vi "Untitled 1.vi"() -> ()   [LabVIEW 2013]
uses:
  <vilib>/Analysis/6fits.llb/Curve Fitting Criteria.ctl
  <vilib>/Analysis/NI_AALPro.lvlib
panel:
  out "XY Graph 3":cluster{"Y":dbl[], "Y":dbl[]}[](graph)
  out "XY Graph 2":cluster{"X":dbl, "Y":dbl}[](graph)
  out "Array":cluster{dbl, dbl}[](array[cluster])
  out "XY Graph":cluster{"X":dbl, "Y":dbl}[](graph)
  in  "Pi/x":dbl
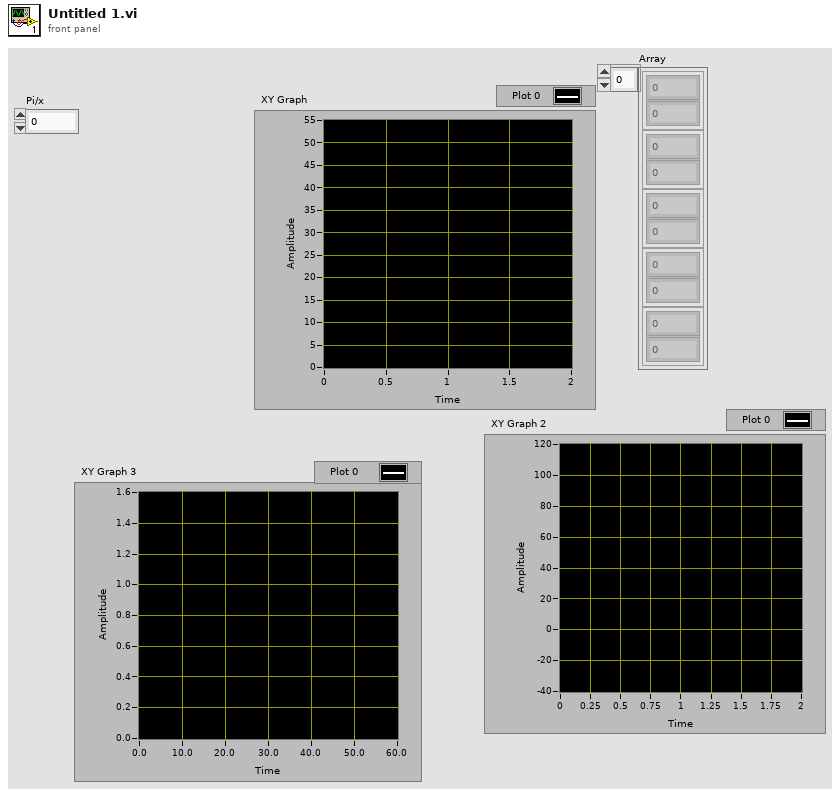
[diagram p1: front panel]
types:
  T1 = typedef "NI_AALPro.lvlib/Curve Fitting Criteria.ctl" = u16
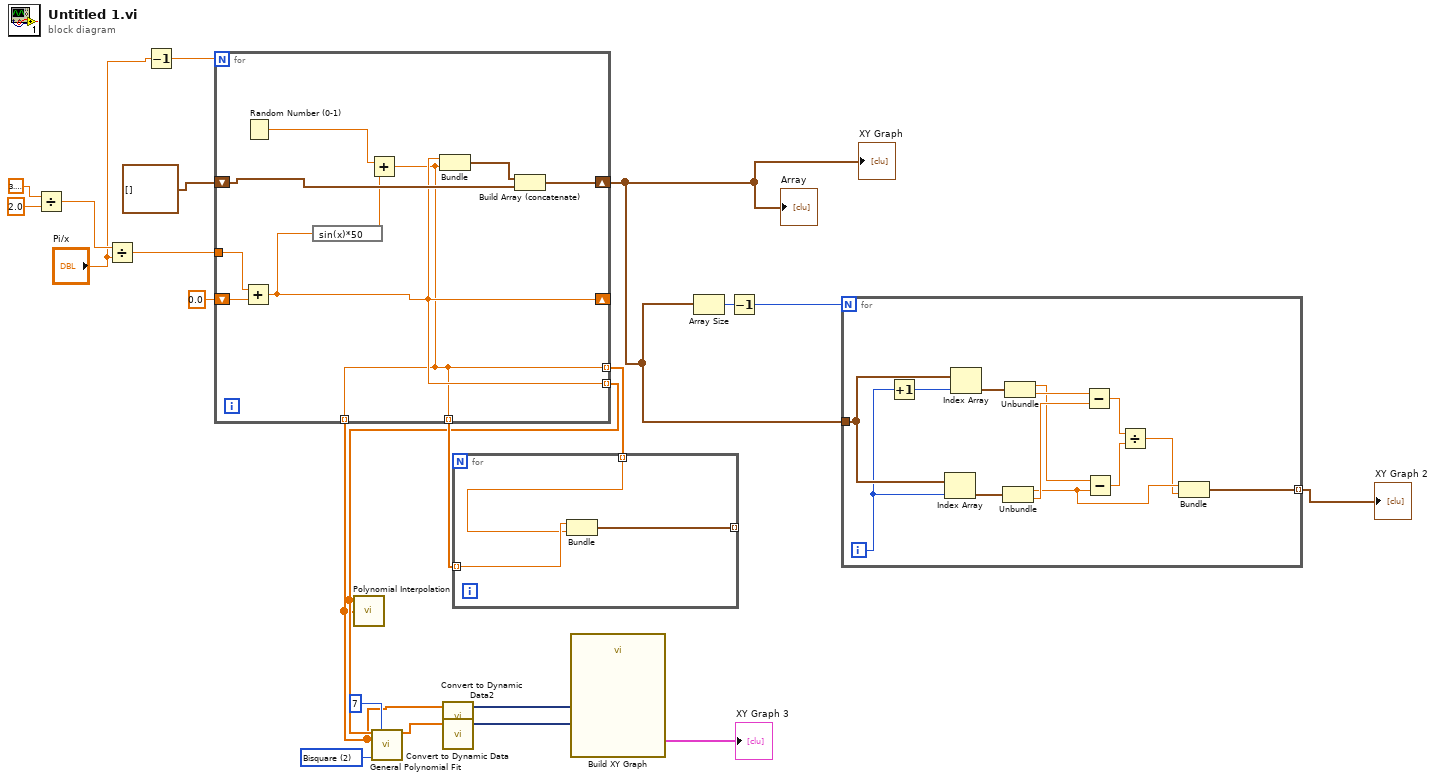
[diagram p0: block diagram]
diagram:
  w6 = T1 2 items=["Least Square", "Least Absolute Residual", "Bisquare"] ("method")
  n1 = Divide(x=3.141592653589793, y=2.0) -> (x/y=w19:dbl)
  n2 = Divide(x=w19, y="Pi/x") -> (x/y=w12:dbl)
  n3 = Decrement(x="Pi/x") -> (x-1=w16:dbl)
  n4 = for {
    N: w16 -> [_]
    tunnel: w12 -> [w31]
    shift-right: [w25] -> _
    shift-left: 0.0 -> [w30]
    shift-right: [w28] -> w1
    shift-left: cluster{dbl, dbl}[] [] -> [w27]
    tunnel: [w25] -> w7 mode=indexing
    tunnel: [w23] -> w4 mode=indexing
    tunnel: [w23] -> w2 mode=indexing
    tunnel: [w23] -> w8 mode=indexing
    n5 = Add(x=w31, y=w30) -> (x+y=w25:dbl)
    n6 = Random Number (0-1)() -> (number: 0 to 1=w24:dbl)
    n7 = expression code="sin(x)*50"(w25) -> (w26:dbl)
    n8 = Add(x=w24, y=w26) -> (x+y=w23:dbl)
    n9 = Bundle(w25, w23) -> (w29:cluster{dbl, dbl})  [unwired: 1 in]
    n10 = Build Array (concatenate)(w29, w27) -> (w28:cluster{dbl, dbl}[])
  }
  "XY Graph" <- w1
  "Array" <- w1
  n11 = call <vilib>:"Polynomial Interpolation.vi"("X"=w2, "Y"=w7) -> ()  [unwired: 1 in, 3 out]
  n12 = call <vilib>:"General Polynomial Fit.vi"("Y"=w7, "polynomial order"=7, "X"=w2, "method"=w6) -> ("Best Polynomial Fit"=w3:dbl[])  [unwired: 8 in, 3 out]
  n13 = call "Convert to Dynamic Data2"("Array"=w2) -> ("Dynamic Data Type"=w9:dynamicdata)  [unwired: 3 in]
  n14 = call "Convert to Dynamic Data"("Array"=w3) -> ("Dynamic Data Type"=w10:dynamicdata)  [unwired: 3 in]
  n15 = for {
    tunnel: w8 -> [w34] mode=indexing
    tunnel: [w33] -> _ mode=indexing
    tunnel: w4 -> [w32] mode=indexing
    n16 = Bundle(w34, w32) -> (w33:cluster{dbl, dbl})  [unwired: 1 in]
  }
  n17 = call "Build XY Graph"("Y Input"=w10, "X Input"=w9) -> ("XY Graph"=→"XY Graph 3":cluster{"X":dbl[], "Y":dbl[]}[])  [unwired: 8 in, 1 out]
  n18 = Array Size(array=w1) -> (size(s)=w15:i32)
  n19 = Decrement(x=w15) -> (x-1=w14:i32)
  n20 = for {
    N: w14 -> [_]
    tunnel: w1 -> [w47]
    tunnel: [w35] -> w13 mode=indexing
    i -> [w44]
    n21 = Increment(x=w44) -> (x+1=w43:i32)
    n22 = Index Array(array=w47, index=w44) -> (element=w45:cluster{dbl, dbl})
    n23 = Index Array(array=w47, index=w43) -> (element=w46:cluster{dbl, dbl})
    n24 = Unbundle(w45) -> (w37:dbl, w41:dbl)
    n25 = Unbundle(w46) -> (w40:dbl, w42:dbl)
    n26 = Subtract(x=w42, y=w41) -> (x-y=w39:dbl)
    n27 = Subtract(x=w40, y=w37) -> (x-y=w38:dbl)
    n28 = Divide(x=w39, y=w38) -> (x/y=w36:dbl)
    n29 = Bundle(w37, w36) -> (w35:cluster{dbl, dbl})  [unwired: 1 in]
  }
  "XY Graph 2" <- w13
